vi "GenerateWave (SubVI).vi"(11 "wave":T1) -> (3 "DC":dynamicdata(waveform))   [LabVIEW 2023]
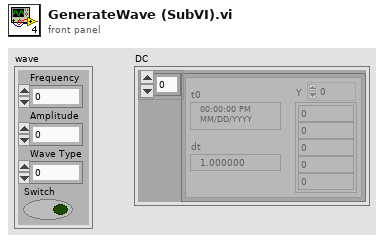
[diagram p1: front panel]
types:
  T1 = cluster{"Frequency":dbl, "Amplitude":dbl, "Wave Type":dbl, "Switch":bool}
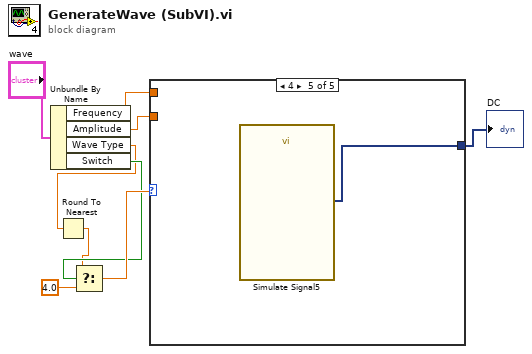
[diagram p0: block diagram]
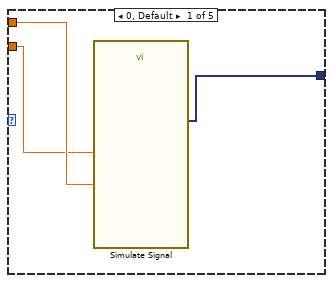
[diagram p2: hidden frame]
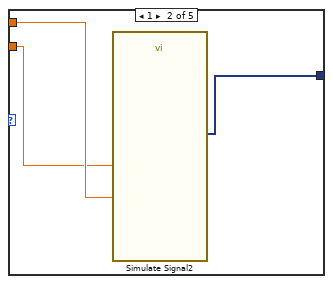
[diagram p3: hidden frame]
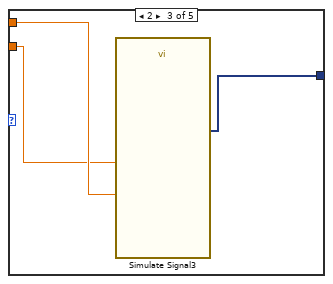
[diagram p4: hidden frame]
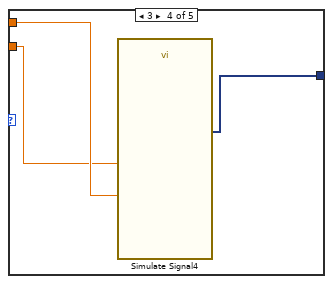
[diagram p5: hidden frame]
diagram:
  n1 = Unbundle By Name("wave") -> ("Frequency"=w3:dbl, "Amplitude"=w2:dbl, "Wave Type"=w1:dbl, "Switch"=w8:bool)
  n2 = Round To Nearest(number=w1) -> (nearest integer value=w7:dbl)
  n3 = Select(t=w7, s=w8, f=4.0) -> (s? t:f=w9:dbl)
  n4 = case shown="4" w9 {
    tunnel: w2 -> [w11 w14 w17 w20 _]
    tunnel: w3 -> [w12 w15 w18 w21 _]
    tunnel: [w10 w13 w16 w19 w22] -> w5
    frame 0, Default {
      n5 = call "Simulate Signal"("Frequency"=w12, "Amplitude"=w11) -> ("Sine"=w10:dynamicdata)  [unwired: 12 in, 1 out]
    }
    frame 1 {
      n6 = call "Simulate Signal2"("Frequency"=w15, "Amplitude"=w14) -> ("Square"=w13:dynamicdata)  [unwired: 12 in, 1 out]
    }
    frame 2 {
      n7 = call "Simulate Signal3"("Frequency"=w18, "Amplitude"=w17) -> ("Triangle"=w16:dynamicdata)  [unwired: 12 in, 1 out]
    }
    frame 3 {
      n8 = call "Simulate Signal4"("Frequency"=w21, "Amplitude"=w20) -> ("Sawtooth"=w19:dynamicdata)  [unwired: 12 in, 1 out]
    }
    frame 4 {
      n9 = call "Simulate Signal5"() -> ("DC"=w22:dynamicdata)  [unwired: 14 in, 1 out]
    }
  }
  "DC" <- w5
